vi "For循环条件接线端.vi"() -> ()   [LabVIEW 2013]
panel:
  out "循环次数":i32
  in  "停止":bool
  out "数字(0-1)":dbl
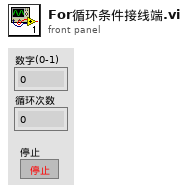
[diagram p1: front panel]
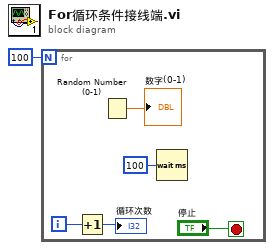
[diagram p0: block diagram]
diagram:
  n1 = for {
    N: 100 -> [_]
    i -> [w3]
    stop <- "停止" stop-if-true
    n2 = Increment(x=w3) -> (x+1=→"循环次数":i32)
    n3 = Random Number (0-1)() -> (number: 0 to 1=→"数字(0-1)":dbl)
    n4 = Wait (ms)(milliseconds to wait=u32 100 ("等待时间（毫秒）")) -> ()  [unwired: 1 out]
  }
